vi "Setup.vi"() -> ()   [LabVIEW 2013]
uses:
  Setup/SetupCtl.ctl
  Model.ctl
  Global.vi
panel:
  in  "Setup":T1
  in  "Cancel":bool
  in  "Save":bool
  in  "Delete":bool
  in  "Flash":bool
  in  "Add":bool
  in  "参数类别":enum16{"设备型号", "上报时间", "电池类型", "软件版本"}(ring)
  in  "设备型号B":u16(ring) items=["TRG80-68"=1, "TRG80-68AW"=2]
  in  "返回":bool
  in  "软件版本E":u16(ring)=1 items=["通用版"=1, "部标版"=2, "神州版"=3, "弘高版"=4]
  in  "电池类型及硬件版本D":u16(ring) items=["无特定电池类型"=0, "松下电池1.0"=1, "GP电池1.0"=3, "松下电池2.0"=5, "GP电池2.0"=7, "其它情况"=9]
  in  "上报时间间隔C":u16(ring) items=["无"=0, "1"=1, "3"=3, "5"=5, "7"=7, "15"=9]
  in  "设备型号A":u16(ring)=1 items=["68有线设备"=1, "68无线设备"=2, "89有线设备"=3, "88无线设备"=4, "90-03系列"=5, "80-03系列"=6]
  in  "选择":enum32{"设备型号", "上报时间", "电池类型", "软件版本"}(tab)
  in  "型号A类型值":string
  in  "型号A类型名":string
  out "设备型号B":string[][](table)
  out "设备型号A":string[][](table)
  out "设备型号AB":string[][](table)
  in  "型号B":string[][](table)
  out "上报时间间隔":string[][](table)
  in  "时间间隔名":string
  in  "时间间隔值":string
  out "电池类型及硬件版本":string[][](table)
  in  "电池类型名":string
  in  "电池类型值":string
  out "软件版本":string[][](table)
  in  "软件版本名":string
  in  "软件版本值":string
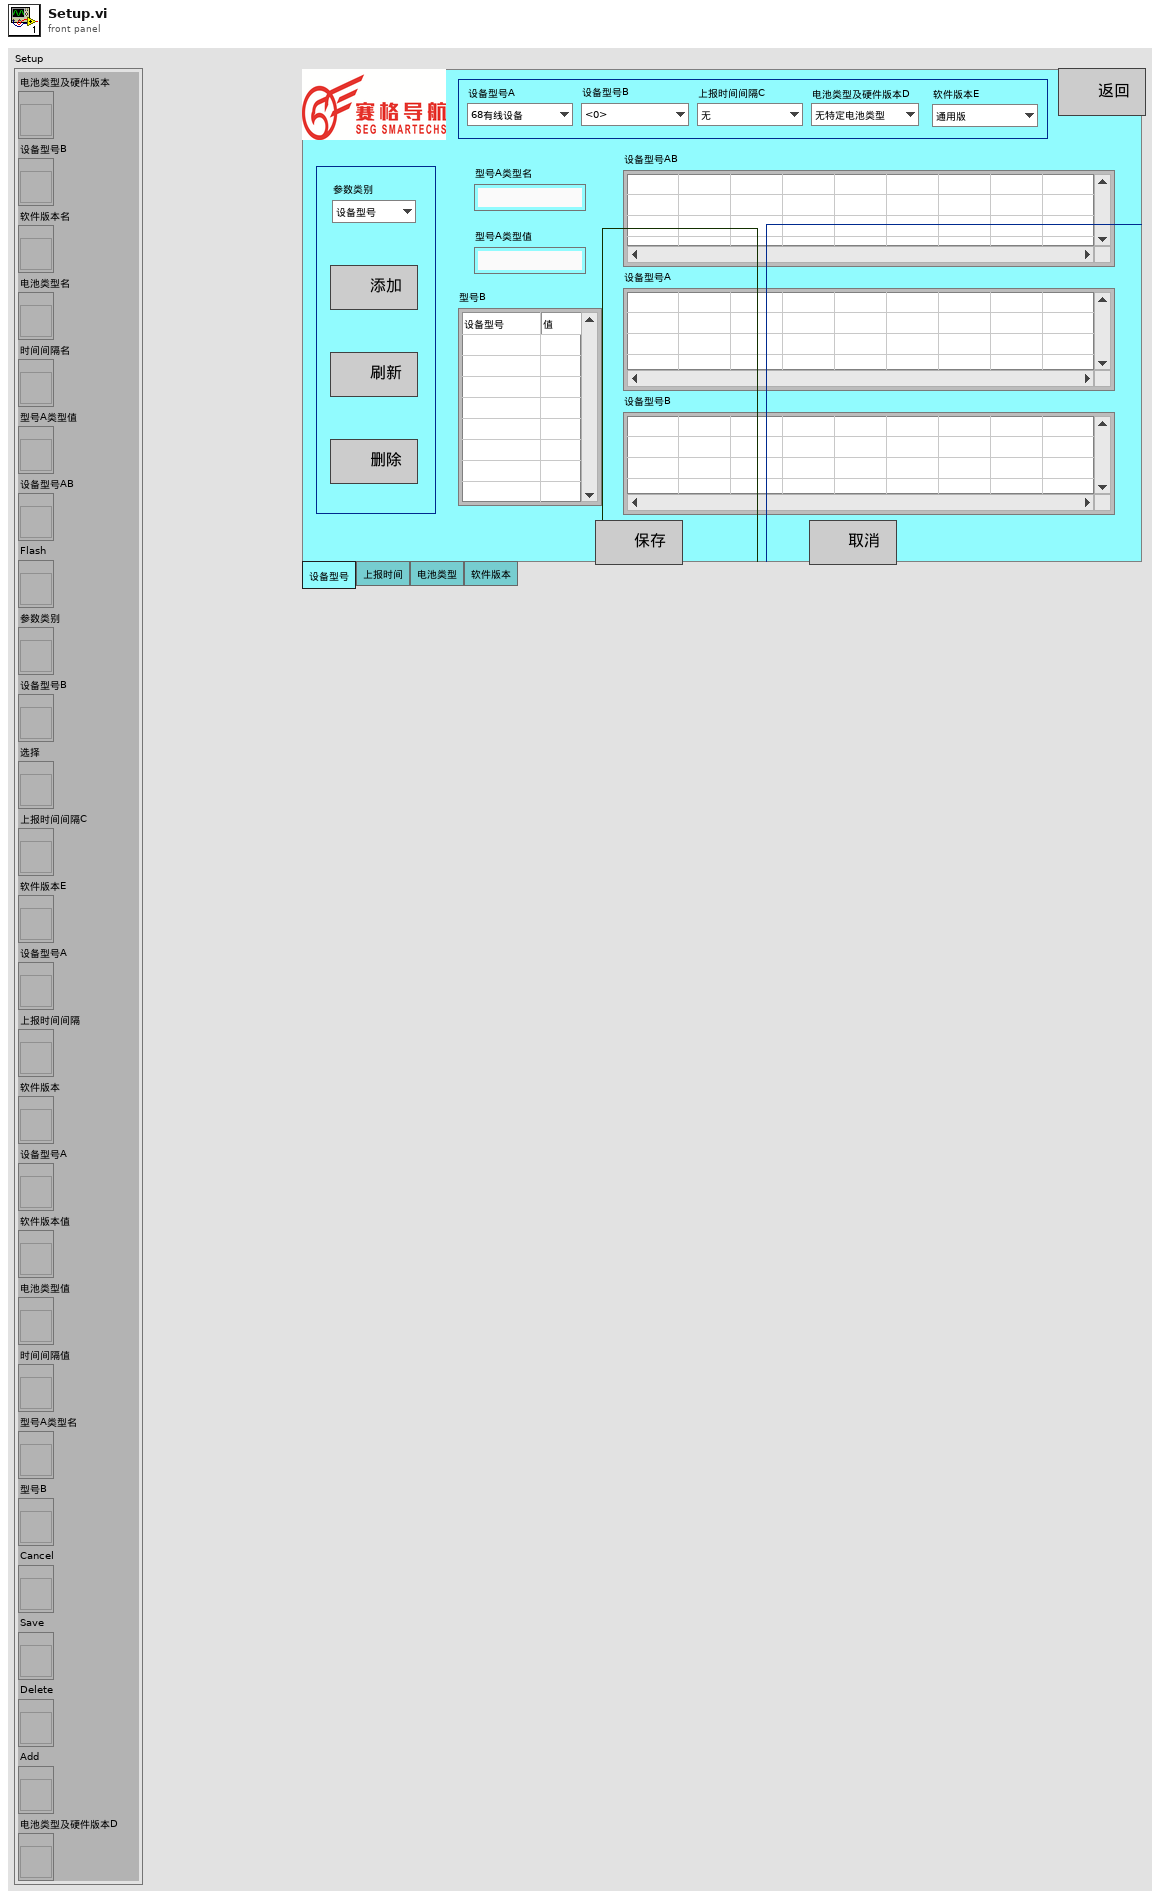
[diagram p1: front panel]
types:
  T1 = typedef "SetupCtl.ctl" = cluster{"电池类型及硬件版本":refnum<vi>, "设备型号B":refnum<vi>, "软件版本名":refnum<vi>, "电池类型名":refnum<vi>, "时间间隔名":refnum<vi>, "型号A类型值":refnum<vi>, "设备型号AB":refnum<vi>, "Flash":refnum<vi>, "参数类别":refnum<vi>, "设备型号B":refnum<vi>, "选择":refnum<vi>, "上报时间间隔C":refnum<vi>, "软件版本E":refnum<vi>, "设备型号A":refnum<vi>, "上报时间间隔":refnum<vi>, "软件版本":refnum<vi>, "设备型号A":refnum<vi>, "软件版本值":refnum<vi>, "电池类型值":refnum<vi>, "时间间隔值":refnum<vi>, "型号A类型名":refnum<vi>, "型号B":refnum<vi>, "Cancel":refnum<vi>, "Save":refnum<vi>, "Delete":refnum<vi>, "Add":refnum<vi>, "电池类型及硬件版本D":refnum<vi>}
  T2 = enum32{"invalid app kind", "Development System", "Run Time System", "Student Edition", "Embedded LabVIEW", "Evaluation", "Custom"}
  T3 = typedef "ParaConfig.ctl" = cluster{"软件版本":string[][], "上报时间间隔":string[][], "电池类型":string[][]}
  T4 = typedef "Model.ctl" = cluster{"AB":string[][], "A":string[][], "B":string[][]}
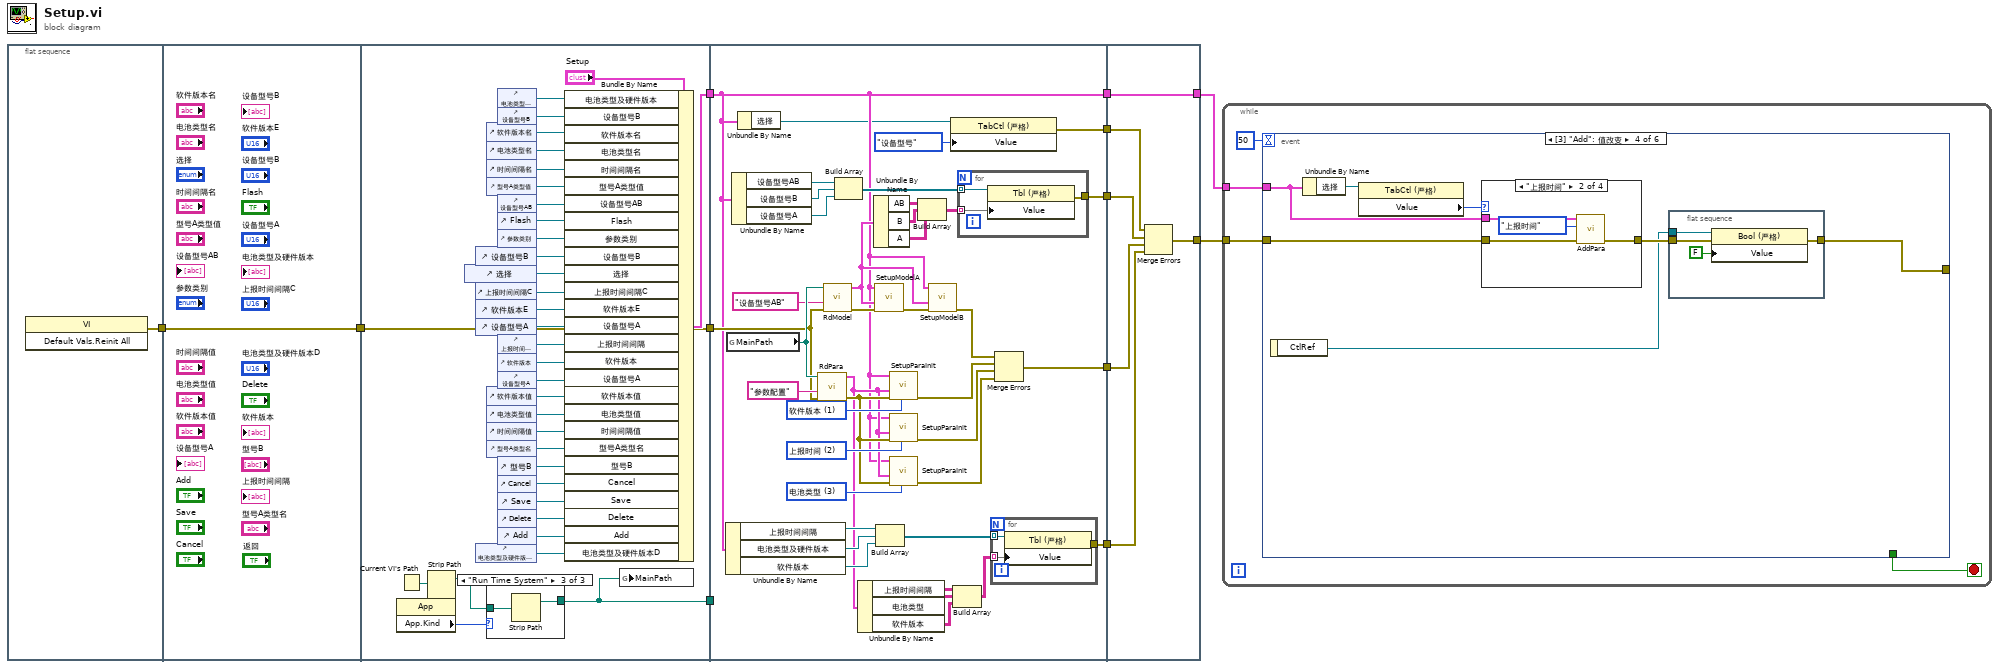
[diagram p0: block diagram]
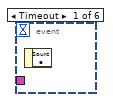
[diagram p4: hidden frame]
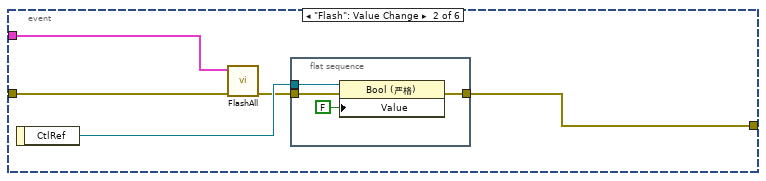
[diagram p5: hidden frame]
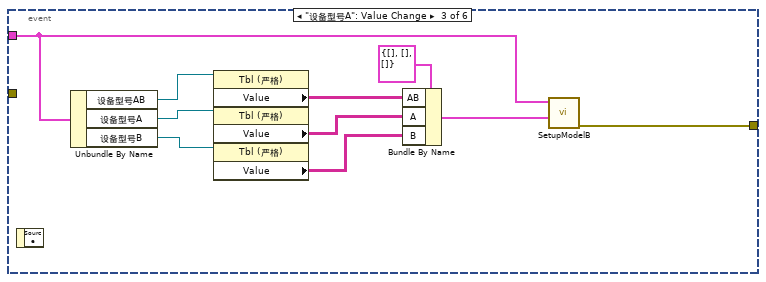
[diagram p6: hidden frame]
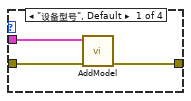
[diagram p7: hidden frame]
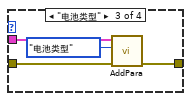
[diagram p8: hidden frame]
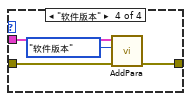
[diagram p9: hidden frame]
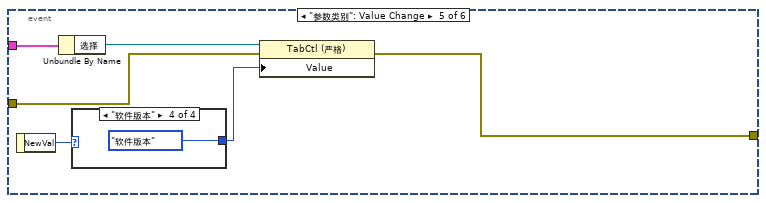
[diagram p10: hidden frame]
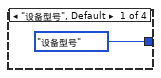
[diagram p11: hidden frame]
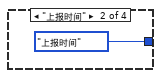
[diagram p12: hidden frame]
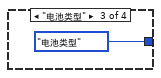
[diagram p13: hidden frame]
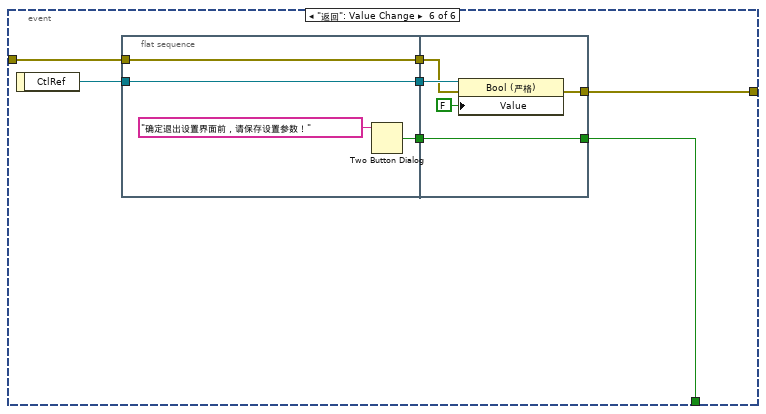
[diagram p14: hidden frame]
diagram:
  n1 = flat-sequence {
    tunnel: [w13] -> w12
    tunnel: w12 -> [w14]
    tunnel: [w14] -> w11
    tunnel: w11 -> [w15]
    tunnel: [w20] -> w10
    tunnel: [w16] -> w9
    tunnel: [w15] -> w8
    tunnel: w10 -> [w58]
    tunnel: w9 -> [_]
    tunnel: w8 -> [w88]
    tunnel: [w58] -> w7
    tunnel: [w77] -> w6
    tunnel: [w55] -> w5
    tunnel: [w54] -> w4
    tunnel: [w53] -> w3
    tunnel: [w103] -> w1
    tunnel: w7 -> [w103]
    tunnel: w6 -> [w100]
    tunnel: w5 -> [w102]
    tunnel: w4 -> [w101]
    tunnel: w3 -> [w99]
    tunnel: [w98] -> w2
    frame #0 {
      n2 = invoke class="VI" method="Default Vals.Reinit All"() -> (error out=w13:errorcluster)  [unwired: 3 in, 2 out]
    }
    frame #1 {
    }
    frame #2 {
      n3 = property class="App"() -> ("App.Kind"=w17:T2)  [unwired: 2 in, 2 out]
      n4 = Current VI's Path() -> (path=w19:path)
      n5 = Strip Path(path=w19) -> (stripped path=w18:path)  [unwired: 1 out]
      n6 = control-ref of="选择"() -> (w37:refnum<vi>)
      n7 = control-ref of="设备型号B"() -> (w38:refnum<vi>)
      n8 = control-ref of="上报时间间隔C"() -> (w36:refnum<vi>)
      n9 = control-ref of="软件版本E"() -> (w35:refnum<vi>)
      n10 = control-ref of="设备型号A"() -> (w34:refnum<vi>)
      n11 = control-ref of="电池类型及硬件版本D"() -> (w21:refnum<vi>)
      n12 = control-ref of="软件版本名"() -> (w45:refnum<vi>)
      n13 = control-ref of="电池类型名"() -> (w44:refnum<vi>)
      n14 = control-ref of="时间间隔名"() -> (w43:refnum<vi>)
      n15 = control-ref of="型号A类型值"() -> (w42:refnum<vi>)
      n16 = control-ref of="软件版本值"() -> (w30:refnum<vi>)
      n17 = control-ref of="电池类型值"() -> (w29:refnum<vi>)
      n18 = control-ref of="时间间隔值"() -> (w28:refnum<vi>)
      n19 = control-ref of="型号A类型名"() -> (w27:refnum<vi>)
      n20 = case shown="\"Run Time System\"" w17 {
        tunnel: w18 -> [w49 w50 w52]
        tunnel: [w49 w50 w51] -> w16
        frame "invalid app kind", Default {
        }
        frame "Development System" {
        }
        frame "Run Time System" {
          n21 = Strip Path(path=w52) -> (stripped path=w51:path)  [unwired: 1 out]
        }
      }
      n22 = control-ref of="电池类型及硬件版本"() -> (w47:refnum<vi>)
      n23 = control-ref of="设备型号B"() -> (w46:refnum<vi>)
      n24 = control-ref of="设备型号AB"() -> (w41:refnum<vi>)
      n25 = control-ref of="Flash"() -> (w40:refnum<vi>)
      n26 = control-ref of="参数类别"() -> (w39:refnum<vi>)
      n27 = control-ref of="上报时间间隔"() -> (w33:refnum<vi>)
      n28 = control-ref of="软件版本"() -> (w32:refnum<vi>)
      n29 = control-ref of="设备型号A"() -> (w31:refnum<vi>)
      n30 = control-ref of="型号B"() -> (w26:refnum<vi>)
      n31 = control-ref of="Cancel"() -> (w25:refnum<vi>)
      n32 = control-ref of="Save"() -> (w24:refnum<vi>)
      n33 = control-ref of="Delete"() -> (w23:refnum<vi>)
      n34 = control-ref of="Add"() -> (w22:refnum<vi>)
      n35 = Bundle By Name(cluster="Setup", "电池类型及硬件版本"=w47, "设备型号B"=w46, "软件版本名"=w45, "电池类型名"=w44, "时间间隔名"=w43, "型号A类型值"=w42, "设备型号AB"=w41, "Flash"=w40, "参数类别"=w39, "设备型号B"=w38, "选择"=w37, "上报时间间隔C"=w36, "软件版本E"=w35, "设备型号A"=w34, "上报时间间隔"=w33, "软件版本"=w32, "设备型号A"=w31, "软件版本值"=w30, "电池类型值"=w29, "时间间隔值"=w28, "型号A类型名"=w27, "型号B"=w26, "Cancel"=w25, "Save"=w24, "Delete"=w23, "Add"=w22, "电池类型及硬件版本D"=w21) -> (w20:T1)
      n36 = global write "Global.vi" "MainPath"(w16) -> ()
    }
    frame #3 {
      w82 = u16 3 items=["软件版本"=1, "上报时间"=2, "电池类型"=3] ("参数选择")
      w84 = u16 2 items=["软件版本"=1, "上报时间"=2, "电池类型"=3] ("参数选择")
      w85 = u16 1 items=["软件版本"=1, "上报时间"=2, "电池类型"=3] ("参数选择")
      n37 = Unbundle By Name(w58) -> ("上报时间间隔"=w67:refnum<vi>, "电池类型及硬件版本"=w66:refnum<vi>, "软件版本"=w65:refnum<vi>)
      n38 = global read "Global.vi" "MainPath"() -> (w90:path)
      n39 = Unbundle By Name(w58) -> ("设备型号AB"=w75:refnum<vi>, "设备型号B"=w74:refnum<vi>, "设备型号A"=w73:refnum<vi>)
      n40 = Unbundle By Name(w58) -> ("选择"=w57:refnum<vi>)
      n41 = call "RdPara.vi"("error in"=w88, "XLSName"="参数配置", "PathIn"=w90) -> ("error out"=w83:errorcluster, "参数配置"=w63:T3)  [unwired: 7 in]
      n42 = call "RdModel.vi"("error in"=w88, "XLSName"="设备型号AB", "PathIn"=w90) -> ("error out"=w87:errorcluster, "设备型号AB"=w76:T4)  [unwired: 7 in]
      n43 = Build Array(w75, w74, w73) -> (w72:refnum<vi>[])
      n44 = Unbundle By Name(w63) -> ("上报时间间隔"=w61:string[][], "电池类型"=w62:string[][], "软件版本"=w60:string[][])
      n45 = Unbundle By Name(w76) -> ("AB"=w71:string[][], "B"=w70:string[][], "A"=w69:string[][])
      n46 = call "SetupModelA.vi"("error in"=w87, "设备型号AB"=w76, "Setup"=w58) -> ("error out"=w86:errorcluster)  [unwired: 8 in]
      n47 = Build Array(w67, w66, w65) -> (w64:refnum<vi>[])
      n48 = call "SetupParaInit.vi"("参数选择"=w85, "error in"=w83, "参数配置"=w63, "Setup"=w58) -> ("error out"=w80:errorcluster)  [unwired: 7 in]
      n49 = call "SetupParaInit.vi"("参数选择"=w84, "error in"=w83, "参数配置"=w63, "Setup"=w58) -> ("error out"=w79:errorcluster)  [unwired: 7 in]
      n50 = call "SetupParaInit.vi"("参数选择"=w82, "error in"=w83, "参数配置"=w63, "Setup"=w58) -> ("error out"=w78:errorcluster)  [unwired: 7 in]
      n51 = Build Array(w71, w70, w69) -> (w68:string[][][])
      n52 = call "SetupModelB.vi"("error in"=w86, "设备型号AB"=w76, "Setup"=w58) -> ("error out"=w81:errorcluster)  [unwired: 8 in]
      n53 = property class="TabCtl (严格)"(reference=w57, "Value"=enum32{"设备型号", "上报时间", "电池类型", "软件版本"}."设备型号" ("值")) -> (error out=w55:errorcluster)  [unwired: 1 in, 1 out]
      n54 = Build Array(w61, w62, w60) -> (w59:string[][][])
      n55 = for {
        tunnel: w72 -> [w97] mode=indexing
        tunnel: w68 -> [w96] mode=indexing
        tunnel: [w95] -> w54
        n56 = property class="Tbl (严格)"(reference=w97, "Value"=w96) -> (error out=w95:errorcluster)  [unwired: 1 in, 1 out]
      }
      n57 = for {
        tunnel: w64 -> [w94] mode=indexing
        tunnel: w59 -> [w93] mode=indexing
        tunnel: [w92] -> w53
        n58 = property class="Tbl (严格)"(reference=w94, "Value"=w93) -> (error out=w92:errorcluster)  [unwired: 1 in, 1 out]
      }
      n59 = Merge Errors(w81, w80, w79, w78) -> (w77:errorcluster)
    }
    frame #4 {
      n60 = Merge Errors(w102, w101, w100, w99) -> (w98:errorcluster)
    }
  }
  n61 = while {
    tunnel: w2 -> [w105]
    tunnel: w1 -> [w104]
    stop <- w107 stop-if-true
    n62 = event shown="[3] \"Add\": 值改变" {
      selector: _ -> [_ _ _ _ _ _]
      dyn-events: _ -> [_ _ _ _ _ _]
      timeout: 50 -> [_ _ _ _ _ _]
      tunnel: [_ _ _ _ _ w167] -> w107
      tunnel: w105 -> [_ w111 _ w130 w154 w169]
      tunnel: [_ w108 w126 w127 w153 w163] -> _
      tunnel: w104 -> [_ w112 w123 w131 w158 _]
      event Timeout {
        n63 = event-data() -> ()  [unwired: 1 in, 1 out]
      }
      event "Flash": Value Change {
        n64 = event-data() -> ("CtlRef"=w110:refnum<vi>)  [unwired: 1 in]
        n65 = call "FlashAll.vi"("error in"=w111, "Setup"=w112) -> ("error out"=w109:errorcluster)  [unwired: 7 in, 2 out]
        n66 = flat-sequence {
          tunnel: w110 -> [w116]
          tunnel: w109 -> [w115]
          tunnel: [w113] -> w108
          frame #0 {
            n67 = property class="Bool (严格)"(reference=w116, error in=w115, "Value"=FALSE ("值")) -> (error out=w113:errorcluster)  [unwired: 1 out]
          }
        }
      }
      event "设备型号A": Value Change {
        n68 = event-data() -> ()  [unwired: 1 in, 1 out]
        n69 = Unbundle By Name(w123) -> ("设备型号AB"=w122:refnum<vi>, "设备型号A"=w120:refnum<vi>, "设备型号B"=w118:refnum<vi>)
        n70 = property class="Tbl (严格)"(reference=w122) -> ("Value"=w121:string[][])  [unwired: 1 in, 2 out]
        n71 = property class="Tbl (严格)"(reference=w120) -> ("Value"=w119:string[][])  [unwired: 1 in, 2 out]
        n72 = property class="Tbl (严格)"(reference=w118) -> ("Value"=w117:string[][])  [unwired: 1 in, 2 out]
        n73 = Bundle By Name(cluster=T4 {"AB"=[], "A"=[], "B"=[]} ("设备型号AB"), "AB"=w121, "A"=w119, "B"=w117) -> (w124:T4)
        n74 = call "SetupModelB.vi"("设备型号AB"=w124, "Setup"=w123) -> ("error out"=w126:errorcluster)  [unwired: 9 in]
      }
      event "Add": Value Change {
        n75 = event-data() -> ("CtlRef"=w128:refnum<vi>)  [unwired: 1 in]
        n76 = Unbundle By Name(w131) -> ("选择"=w133:refnum<vi>)
        n77 = property class="TabCtl (严格)"(reference=w133) -> ("Value"=w132:enum32{"设备型号", "上报时间", "电池类型", "软件版本"})  [unwired: 1 in, 2 out]
        n78 = case shown="\"上报时间\"" w132 {
          tunnel: w131 -> [w140 w144 w148 w152]
          tunnel: w130 -> [w139 w143 w147 w151]
          tunnel: [w138 w141 w145 w149] -> w129
          frame "设备型号", Default {
            n79 = call "AddModel.vi"("error in"=w139, "Setup"=w140) -> ("error out"=w138:errorcluster)  [unwired: 9 in]
          }
          frame "上报时间" {
            n80 = call "AddPara.vi"("error in"=w143, "选择"=enum16{"上报时间", "电池类型", "软件版本"}."上报时间", "Setup"=w144) -> ("error out"=w141:errorcluster)  [unwired: 8 in]
          }
          frame "电池类型" {
            n81 = call "AddPara.vi"("error in"=w147, "选择"=enum16{"上报时间", "电池类型", "软件版本"}."电池类型", "Setup"=w148) -> ("error out"=w145:errorcluster)  [unwired: 8 in]
          }
          frame "软件版本" {
            n82 = call "AddPara.vi"("error in"=w151, "选择"=enum16{"上报时间", "电池类型", "软件版本"}."软件版本", "Setup"=w152) -> ("error out"=w149:errorcluster)  [unwired: 8 in]
          }
        }
        n83 = flat-sequence {
          tunnel: w129 -> [w136]
          tunnel: w128 -> [w137]
          tunnel: [w135] -> w127
          frame #0 {
            n84 = property class="Bool (严格)"(reference=w137, error in=w136, "Value"=FALSE ("值")) -> (error out=w135:errorcluster)  [unwired: 1 out]
          }
        }
      }
      event "参数类别": Value Change {
        n85 = event-data() -> ("NewVal"=w156:enum16{"设备型号", "上报时间", "电池类型", "软件版本"})  [unwired: 1 in]
        n86 = Unbundle By Name(w158) -> ("选择"=w157:refnum<vi>)
        n87 = case shown="\"软件版本\"" w156 {
          tunnel: [enum32{"设备型号", "上报时间", "电池类型", "软件版本"}."设备型号" ("值") enum32{"设备型号", "上报时间", "电池类型", "软件版本"}."上报时间" ("值") enum32{"设备型号", "上报时间", "电池类型", "软件版本"}."电池类型" ("值") enum32{"设备型号", "上报时间", "电池类型", "软件版本"}."软件版本" ("值")] -> w155
          frame "设备型号", Default {
          }
          frame "上报时间" {
          }
          frame "电池类型" {
          }
          frame "软件版本" {
          }
        }
        n88 = property class="TabCtl (严格)"(reference=w157, error in=w154, "Value"=w155) -> (error out=w153:errorcluster)  [unwired: 1 out]
      }
      event "返回": Value Change {
        n89 = event-data() -> ("CtlRef"=w168:refnum<vi>)  [unwired: 1 in]
        n90 = flat-sequence {
          tunnel: w169 -> [w171]
          tunnel: w168 -> [w170]
          tunnel: [w172] -> w166
          tunnel: [w171] -> w165
          tunnel: [w170] -> w164
          tunnel: [w178] -> w167
          tunnel: w166 -> [w178]
          tunnel: w165 -> [w175]
          tunnel: w164 -> [w177]
          tunnel: [w174] -> w163
          frame #0 {
            n91 = Two Button Dialog(message="确定退出设置界面前，请保存设置参数！" ("消息")) -> (T button?=w172:bool)  [unwired: 2 in]
          }
          frame #1 {
            n92 = property class="Bool (严格)"(reference=w177, error in=w175, "Value"=FALSE ("值")) -> (error out=w174:errorcluster)  [unwired: 1 out]
          }
        }
      }
    }
  }
